vi "Close Async.vi"(8 "error in (no error)":errorcluster, 10 "Event Registration":refnum<event-registration>, 11 "Async Data":T1) -> (0 "error out":errorcluster)   [LabVIEW 2012, in "Waveform Data Logger Engine.lvlib"]
uses:
  Waveform Data Logger Engine.lvlib
  Types/Async Data.ctl
  <vilib>/NI Veristand/Custom Device Waveform API/Multiple Waveforms Read (DBL)/Multiple Waveforms Read (DBL).lvclass
  Classes/Waveforms/Utilities/Reference Dictionary/Reference Dictionary.lvclass
  Types/Wfm Acq Data.ctl
  Classes/Waveforms/Waveform Receive/Waveform Receive.lvclass
  Classes/Waveforms/Waveform Log/Waveform Log.lvclass
  Types/Async Communication.ctl
  Types/Check File Loop Cmd.ctl
  Types/Trigger Event Data.ctl
  Types/Trigger Received.ctl
  Types/New File Event Data.ctl
  <vilib>/NI Veristand/Custom Device Waveform API/Multiple Waveforms Read (DBL)/NI VeriStand - Close Multiple Waveforms Read Session (DBL).vi
  <userlib>/_OpenG.lib/error/error.llb/Filter Error Codes (Array)__ogtk.vi
  <vilib>/NI VeriStand/Custom Device Waveform API/NI_VS Custom Device Waveform API.lvlib
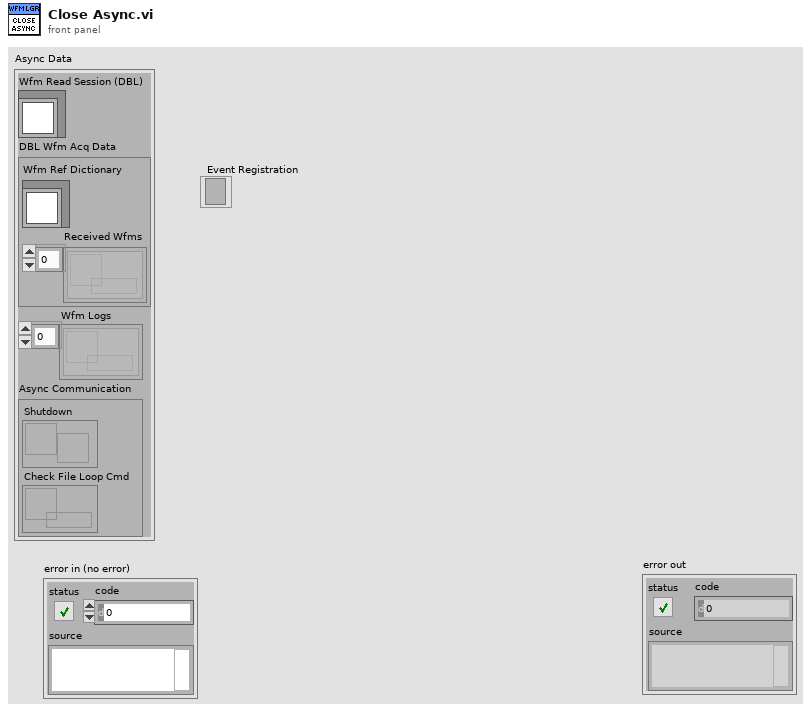
[diagram p1: front panel]
types:
  T1 = typedef "Waveform Data Logger Engine.lvlib/Async Data.ctl" = cluster{"Wfm Read Session (DBL)":refnum<class "Multiple Waveforms Read (DBL).lvclass">, "DBL Wfm Acq Data":T2, "Wfm Logs":refnum<data-value>[], "Async Communication":T3}
  T2 = typedef "Waveform Data Logger Engine.lvlib/Wfm Acq Data.ctl" = cluster{"Wfm Ref Dictionary":refnum<class "Reference Dictionary.lvclass">, "Received Wfms":refnum<data-value>[]}
  T3 = typedef "Waveform Data Logger Engine.lvlib/Async Communication.ctl" = cluster{"Shutdown":refnum<user-event>, "Check File Loop Cmd":refnum<queue>}
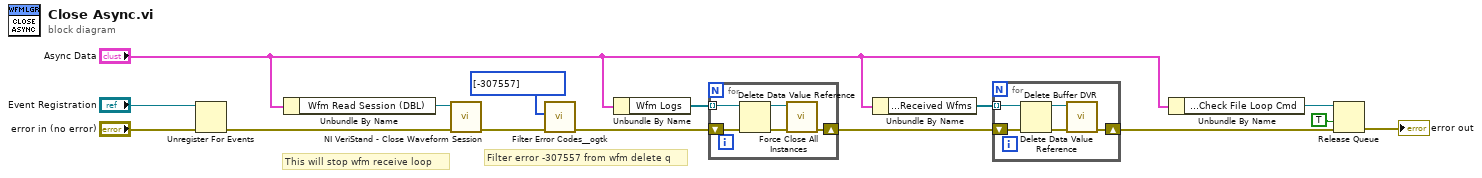
[diagram p0: block diagram]
diagram:
  # "Filter error -307557 from wfm delete q"
  # "This will stop wfm receive loop"
  n1 = Unregister For Events(event registration refnum="Event Registration", error in="error in (no error)") -> (error out=w5:errorcluster)
  n2 = Unbundle By Name("Async Data") -> ("Wfm Read Session (DBL)"=w15:refnum<class "Multiple Waveforms Read (DBL).lvclass">)
  n3 = call-poly <vilib>:"NI VeriStand - Close Waveform Session.vi"("error in (no error)"=w5, "Multiple Waveforms Read Session (DBL)"=w15) -> ("error out"=w2:errorcluster)  [unwired: 9 in]
  n4 = call-poly <userlib>:"Filter Error Codes__ogtk.vi"("Error In"=w2, "Error Codes to Filter"=i32[] [-307557]) -> ("Error Out"=w1:errorcluster)  [unwired: 7 in, 2 out]
  n5 = Unbundle By Name("Async Data") -> ("Wfm Logs"=w14:refnum<data-value>[])
  n6 = for {
    tunnel: w14 -> [w20] mode=indexing
    shift-right: [w16] -> w12
    shift-left: w1 -> [w19]
    n7 = Delete Data Value Reference(data value reference=w20, error in=w19) -> (data value=w17:refnum<class "Waveform Log.lvclass">, error out=w18:errorcluster)
    n8 = call "Force Close All Instances.vi"("error in (no error)"=w18, "Waveform Log in"=w17) -> ("error out"=w16:errorcluster)  [unwired: 9 in]
  }
  n9 = Unbundle By Name("Async Data") -> ("DBL Wfm Acq Data.Received Wfms"=w13:refnum<data-value>[])
  n10 = for {
    tunnel: w13 -> [w25] mode=indexing
    shift-right: [w21] -> w10
    shift-left: w12 -> [w24]
    n11 = Delete Data Value Reference(data value reference=w25, error in=w24) -> (data value=w23:refnum<class "Waveform Receive.lvclass">, error out=w22:errorcluster)
    n12 = call "Delete Buffer DVR.vi"("error in (no error)"=w22, "Waveform Receive in"=w23) -> ("error out"=w21:errorcluster)  [unwired: 9 in]
  }
  n13 = Unbundle By Name("Async Data") -> ("Async Communication.Check File Loop Cmd"=w11:refnum<queue>)
  n14 = Release Queue(queue=w11, force destroy? (F)=TRUE, error in (no error)=w10) -> (error out=→"error out":errorcluster)  [unwired: 2 out]
